vi "Texture Defect Detection.vi"() -> ()   [LabVIEW 2016]
doc: "This example shows how to use the texture defect detection VI in NI Vision.\n\nTexture defect detection identifies areas of the image presentating a significantly different texture. First, use the Texture Training Interface to teach your application a reference texture. The Texture Training Interface creates a texture classifier file, which you then use to detect texture defects."
uses:
  <vilib>/vision/NI_Vision_Development_Module.lvlib
panel:
  out "Number of Defects":i32
  in  "Stop":bool
  in  "Delay (s.)":dbl(slide)=1.008 scale=0.0..2.0
  out "Image":T1(plugin-control)
  # "Overview: Demonstrates detecting texture defects.\nRequirements: NI Vision Development Module\nInstructions: Run the VI and check out the defects found by program."
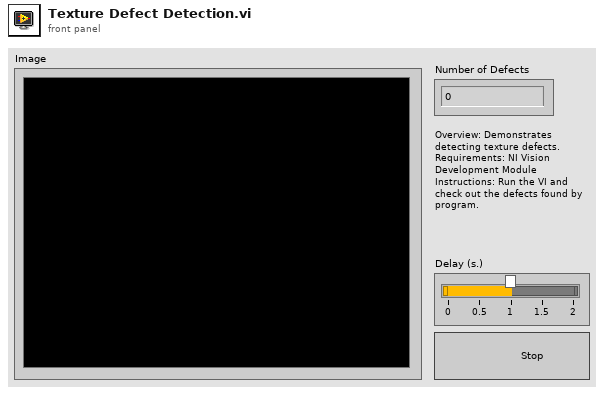
[diagram p1: front panel]
types:
  T1 = typedef "IMAQ Image.ctl" = refnum<image>
  T2 = typedef "IMAQ Classifier Session.ctl" = refnum<k1>
  T3 = typedef "ROI Descriptor" = cluster{"Global Rectangle":i32[], "Contours":cluster{"ID":enum32{"External", "Internal"}, "Type":u32, "Coordinates":i32[]}[]}
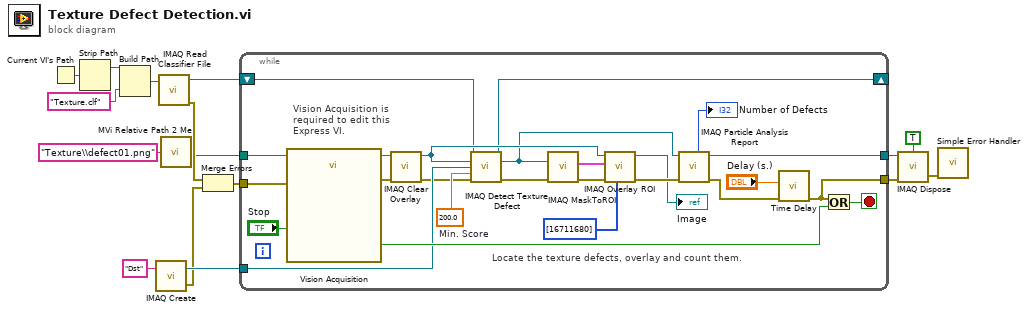
[diagram p0: block diagram]
diagram:
  n1 = Current VI's Path() -> (path=w13:path)
  n2 = Strip Path(path=w13) -> (stripped path=w14:path)  [unwired: 1 out]
  n3 = Build Path(base path=w14, name or relative path="Texture.clf") -> (appended path=w12:path)
  n4 = call "IMAQ Create"("Image Name"="Dst") -> ("Src"=w9:T1, "error out"=w6:errorcluster)  [unwired: 3 in, 1 out]
  n5 = call "IMAQ Read Classifier File"("File Path"=w12) -> ("error out"=w7:errorcluster, "Classifier Session"=w8:T2)  [unwired: 3 in, 6 out]
  n6 = call "MVi Relative Path 2 Me.vi"("Relative Path"="Texture\\defect01.png" ("name or relative path")) -> ("Appended Dir"=w3:path)  [unwired: 5 in, 1 out]
  n7 = Merge Errors(w7, w6) -> (w5:errorcluster)
  n8 = while {
    tunnel: w3 -> [w39]
    tunnel: [w25] -> w16
    tunnel: [w35] -> w15
    tunnel: w9 -> [w21]
    shift-right: [w23] -> _
    shift-left: w8 -> [w24]
    tunnel: w5 -> [w19]
    stop <- w36 stop-if-true
    w34 = 200.0  # Min. Score
    # "Vision Acquisition is required to edit this Express VI."
    # "Locate the texture defects, overlay and count them."
    n9 = call "Vision Acquisition"("Image Path"=w39, "Stop (F)"="Stop", "error in"=w19) -> ("Image Out"=w22:T1, "Stopped"=w37:bool, "error out"=w38:errorcluster)  [unwired: 22 in]
    n10 = call "IMAQ Clear Overlay"("error in (no error)"=w38, "Image"=w22) -> ("error out"=w20:errorcluster, "Image Out"=w28:T1)  [unwired: 1 in, 7 out]
    n11 = call "IMAQ Detect Texture Defect"("Classifier Session"=w24, "Image Src"=w28, "Image Dst"=w21, "Min. Defect Identification Score"=w34, "error in (no error)"=w20) -> ("Classifier Session (dup)"=w23:T2, "Image Dst Out"=w18:T1, "error out"=w29:errorcluster)  [unwired: 4 in, 4 out]
    n12 = call "IMAQ MaskToROI"("Image"=w18, "error in (no error)"=w29) -> ("ROI Descriptor"=w31:T3, "error out"=w30:errorcluster)  [unwired: 2 in, 4 out]
    n13 = call "IMAQ Overlay ROI"("Colors (Green)"=u32[] [16711680], "error in (no error)"=w30, "ROI Descriptor"=w31, "Image"=w28) -> ("error out"=w33:errorcluster, "Image Out"=→"Image":T1)  [unwired: 2 in, 4 out]
    n14 = call "IMAQ Particle Analysis Report"("error in (no error)"=w33, "Image"=w18) -> ("error out"=w27:errorcluster, "Image Out (duplicate)"=w25:T1, "Number of Particles"=→"Number of Defects":i32)  [unwired: 1 in, 6 out]
    n15 = call "Time Delay"("error in (no error)"=w27, "Delay Time (s)"="Delay (s.)") -> ("error out"=w35:errorcluster)  [unwired: 9 in]
    n16 = Or(x=w35, y=w37) -> (x .or. y?=w36:bool)
  }
  n17 = call "IMAQ Dispose"("All Images? (No)"=TRUE, "Image"=w16, "error in (no error)"=w15) -> ("error out"=w1:errorcluster)  [unwired: 3 out]
  n18 = call <vilib>:"Simple Error Handler.vi"("error in (no error)"=w1) -> ()  [unwired: 4 in, 5 out]
